vi "Trigger LEDs.vi"(7 "Trigger":T1={"Mode"=enum."Laser (TAS)", "Source "=enum."Channel 1", "PIA"={"Test LEDs"=FALSE, "LED line"="", "LED off (s)"=0.0, "LED on (s)"=0.0}, "Threshold (V)"=0.0004} {"Threshold (V)" format="%#_3f"}, 8 "error in (no error)":errorcluster) -> (0 "error out":errorcluster)   [LabVIEW 2017, in "Scope.lvlib" / "Trigger.lvlib"]
uses:
  Trigger/Trigger.lvlib
  Trigger/Controls/Params.ctl
  Trigger/Controls/Mode.ctl
  Trigger/Controls/Trigger channels.ctl
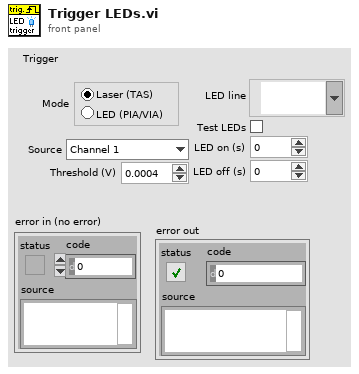
[diagram p1: front panel]
types:
  T1 = typedef "Scope.lvlib/Trigger.lvlib/Params.ctl" = cluster{"Mode":T2, "Source ":T3, "PIA":cluster{"Test LEDs":bool, "LED line":tag, "LED off (s)":dbl, "LED on (s)":dbl}, "Threshold (V)":dbl}
  T2 = typedef "Scope.lvlib/Trigger.lvlib/Mode.ctl" = enum32{"Laser (TAS)", "LED (PIA/VIA)"}
  T3 = typedef "Scope.lvlib/Trigger.lvlib/Trigger channels.ctl" = enum16{"Channel 1", "Channel 2", "Channel 3", "Channel 4", "AC Line", "Aux", "Digital Channel 0", "Digital Channel 1", "Digital Channel 2", "Digital Channel 3", "Digital Channel 4", "Digital Channel 5", "Digital Channel 6", "Digital Channel 7", "Digital Channel 8", "Digital Channel 9", "Digital Channel 10", "Digital Channel 11", "Digital Channel 12", "Digital Channel 13", "Digital Channel 14", "Digital Channel 15", "RF"}
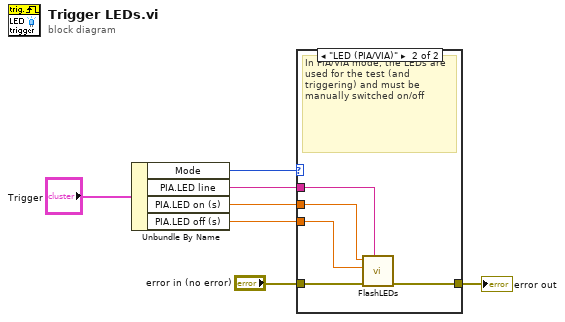
[diagram p0: block diagram]
diagram:
  n1 = Unbundle By Name("Trigger") -> ("Mode"=w6:T2, "PIA.LED line"=w5:tag, "PIA.LED on (s)"=w4:dbl, "PIA.LED off (s)"=w3:dbl)
  n2 = case shown="\"LED (PIA/VIA)\"" w6 {
    tunnel: [w8 w13] -> w1
    tunnel: w5 -> [_ w9]
    tunnel: w4 -> [_ w12]
    tunnel: w3 -> [_ w11]
    tunnel: "error in (no error)" -> [w8 w10]
    frame "Laser (TAS)", Default {
    }
    frame "LED (PIA/VIA)" {
      # "In PIA/VIA mode, the LEDs are used for the test (and triggering) and must be manually switched on/off"
      n3 = call "FlashLEDs.vi"("LED line"=w9, "error in (no error)"=w10, "LED off (s)"=w11, "LED on (s)"=w12) -> ("error out"=w13:errorcluster)  [unwired: 7 in]
    }
  }
  "error out" <- w1
